vi "getSize.vi"(8 "error in (no error)":errorcluster, 11 "ILogFileInfo in":refnum<class "ILogFileInfo.lvclass">) -> (0 "error out":errorcluster, 2 "Size out":i32, 3 "ILogFileInfo out":refnum<class "ILogFileInfo.lvclass">)   [LabVIEW 2022 SP3, in "openDAQ.lvlib" / "IBaseObject.lvlib" / "ILogFileInfo.lvlib" / "ILogFileInfo.lvclass"]
uses:
  <instrlib>/openDAQ/Public/Classes/ILogFileInfo/ILogFileInfo.lvclass
  <instrlib>/openDAQ/Public/Classes/ILogFileInfo/ILogFileInfo.lvclass/ILogFileInfo.ctl
  <instrlib>/openDAQ/Binaries/Windows/x86/copendaq32.dll
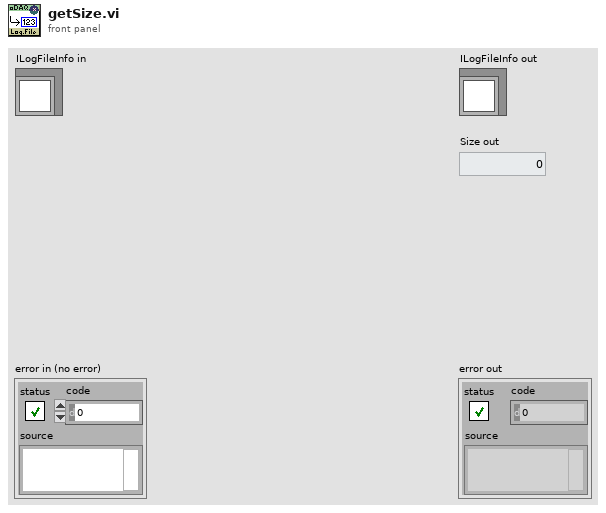
[diagram p1: front panel]
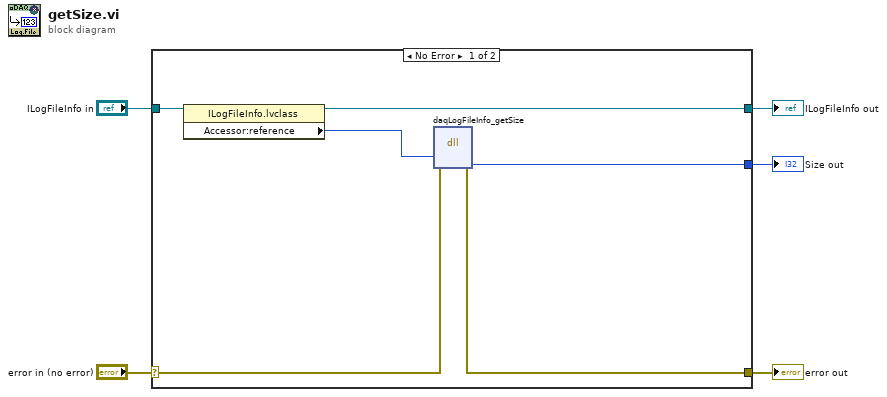
[diagram p0: block diagram]
diagram:
  n1 = case shown="No Error" "error in (no error)" {
    selector: "error in (no error)" -> [w8 w14]
    tunnel: [w7 w14] -> w4
    tunnel: [w10 w13] -> w2
    tunnel: "ILogFileInfo in" -> [w11 w13]
    tunnel: [w6 w12] -> w1
    frame No Error {
      n2 = property class="ILogFileInfo.lvclass"(reference=w11) -> (reference out=w10:refnum<class "ILogFileInfo.lvclass">, "Accessor:reference"=w9:i64)  [unwired: 1 in, 1 out]
      n3 = dll-call lib="C:/Program Files (x86)/National Instruments/LabVIEW 2022/instr.lib/openDAQ/Binaries/Windows/x86/copendaq*.*" fn="daqLogFileInfo_getSize"(error in=w8, "logFileInfo"=w9) -> (error out=w7:errorcluster, "size"=w6:i32)  [unwired: 5 in, 1 out]
    }
    frame Error {
    }
  }
  "error out" <- w4
  "ILogFileInfo out" <- w2
  "Size out" <- w1
